vi "Cube Root of XiXi-1.vi"(10 "X[-1]":dbl, 11 "Xi":dbl[](array[numeric])) -> (3 "Yi":dbl[](array[numeric]) format="%.2f")   [LabVIEW 2011]
doc: "Calculate sums of consecutive array elements. 0th element of output is equal to x(0)+ x(-1), where x(-1) is an optional scalar input that defaults to zero."
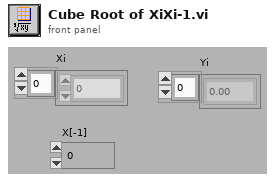
[diagram p1: front panel]
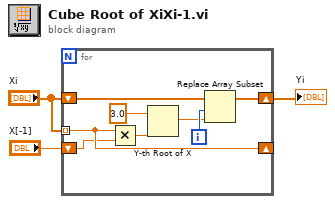
[diagram p0: block diagram]
diagram:
  n1 = for {
    shift-right: [w10] -> w1
    shift-left: "Xi" -> [w11]
    shift-right: [w7] -> _
    shift-left: "X[-1]" -> [w6]
    tunnel: "Xi" -> [w7] mode=indexing
    i -> [w9]
    n2 = Multiply(x=w7, y=w6) -> (x*y=w8:dbl)
    n3 = Y-th Root of X(1:w8, 2:3.0 ("y")) -> (0:w5:dbl)
    n4 = Replace Array Subset(array=w11, new element=w5, index=w9) -> (w10:dbl[])
  }
  "Yi" <- w1
